vi "DBL-to-IEEE754.vi"(11 "Input_DBL":dbl(slide) scale=-20.0..20.0) -> (3 "Output_U8":u8[](array[numeric]))   [LabVIEW 2017]
panel:
  out "Array":bool[][](array[boolean])
  out "appended array":bool[](array[boolean])
  out "Sign":bool=TRUE
  out "Mantissa":bool[](array[boolean])=[TRUE, FALSE, FALSE, TRUE, FALSE, TRUE, FALSE, FALSE, FALSE, TRUE, TRUE, FALSE, FALSE, TRUE, TRUE, TRUE, FALSE, TRUE, TRUE, FALSE, TRUE, TRUE, FALSE]
  out "Exponent":bool[](array[boolean])=[TRUE, FALSE, FALSE, FALSE, FALSE, TRUE, FALSE, TRUE]
  out "Number":dbl=-101.10099792480469 format="%.12f"
  out "Exponent 2":dbl=6.0 format="%.2f"
  out "Mantissa 2":dbl=1.5797030925750732 format="%.8f"
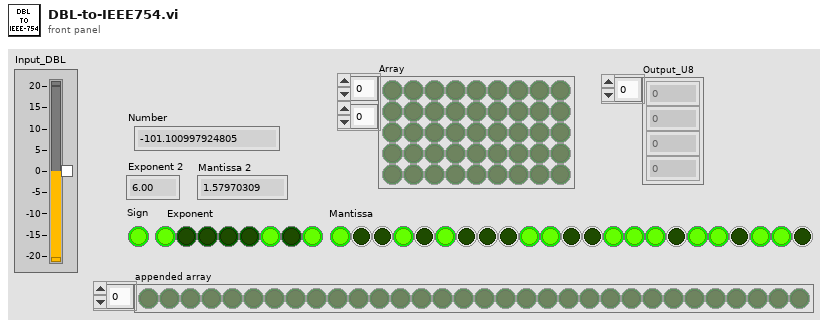
[diagram p1: front panel]
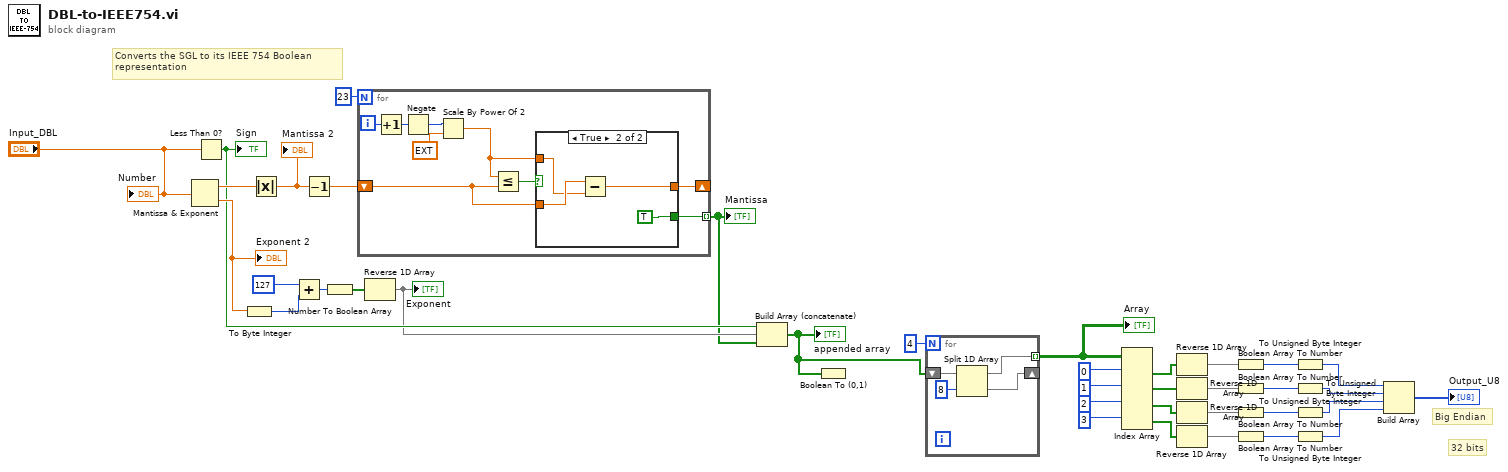
[diagram p0: block diagram]
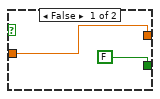
[diagram p2: hidden frame]
diagram:
  # "32 bits"
  # "Big Endian"
  # "Converts the SGL to its IEEE 754 Boolean \nrepresentation"
  n1 = Mantissa & Exponent(0:"Input_DBL") -> (1:w29:dbl, 2:w31:dbl)
  "Exponent 2" <- w31
  n2 = Less Than 0?(x="Input_DBL") -> (x < 0?=w28:bool)
  "Sign" <- w28
  n3 = To Byte Integer(number=w31) -> (8bit integer=w37:i8)
  n4 = Absolute Value(x=w29) -> (abs(x)=w30:dbl)
  "Mantissa 2" <- w30
  n5 = Add(x=i8 127, y=w37) -> (x+y=w36:i8)
  n6 = Decrement(x=w30) -> (x-1=w33:dbl)
  n7 = Number To Boolean Array(number=w36) -> (Boolean array=w35:bool[])
  n8 = for {
    N: 23 -> [_]
    shift-right: [w39] -> _
    shift-left: w33 -> [w41]
    tunnel: [w38] -> w26 mode=indexing
    i -> [w46]
    n9 = Increment(x=w46) -> (x+1=w45:i32)
    n10 = Negate(x=w45) -> (-x=w44:i32)
    n11 = Scale By Power Of 2(n=w44, x=ext 1.0) -> (x*2^n=w40:ext)
    n12 = Less Or Equal?(x=w40, y=w41) -> (x <= y?=w42:bool)
    n13 = case shown="True" w42 {
      tunnel: w41 -> [w47 w52]
      tunnel: w40 -> [_ w49]
      tunnel: [w47 w51] -> w39
      tunnel: [FALSE TRUE] -> w38
      frame False {
      }
      frame True {
        n14 = Subtract(x=w52, y=w49) -> (x-y=w51:ext)
      }
    }
  }
  "Mantissa" <- w26
  n15 = Reverse 1D Array(array=w35) -> (reversed array=w27:bool[])
  "Exponent" <- w27
  n16 = Build Array (concatenate)(w28, w27, w26) -> (w24:bool[])
  "appended array" <- w24
  n17 = Boolean To (0,1)(Boolean=w24) -> ()  [unwired: 1 out]
  n18 = for {
    N: 4 -> [_]
    shift-right: [w55] -> _
    shift-left: w24 -> [w56]
    tunnel: [w54] -> w23 mode=indexing
    n19 = Split 1D Array(array=w56, index=8) -> (first subarray=w54:bool[], second subarray=w55:bool[])
  }
  "Array" <- w23
  n20 = Index Array(array=w23, index (row) #1=0 ("disabled index (col)"), index (row) #2=1 ("index (col)"), index (row) #3=2 ("index (col)"), index (row) #4=3 ("index (col)")) -> (element #1=w4:bool[], element #2=w3:bool[], element #3=w2:bool[], element #4=w1:bool[])  [unwired: 4 in]
  n21 = Reverse 1D Array(array=w4) -> (reversed array=w8:bool[])
  n22 = Reverse 1D Array(array=w3) -> (reversed array=w7:bool[])
  n23 = Reverse 1D Array(array=w2) -> (reversed array=w6:bool[])
  n24 = Reverse 1D Array(array=w1) -> (reversed array=w5:bool[])
  n25 = Boolean Array To Number(Boolean array=w8) -> (number=w18:u32)
  n26 = Boolean Array To Number(Boolean array=w7) -> (number=w17:u32)
  n27 = Boolean Array To Number(Boolean array=w6) -> (number=w16:u32)
  n28 = Boolean Array To Number(Boolean array=w5) -> (number=w15:u32)
  n29 = To Unsigned Byte Integer(number=w18) -> (unsigned 8bit integer=w12:u8)
  n30 = To Unsigned Byte Integer(number=w17) -> (unsigned 8bit integer=w11:u8)
  n31 = To Unsigned Byte Integer(number=w16) -> (unsigned 8bit integer=w10:u8)
  n32 = To Unsigned Byte Integer(number=w15) -> (unsigned 8bit integer=w9:u8)
  n33 = Build Array(w12, w11, w10, w9) -> (→"Output_U8":u8[])
  "Number" <- "Input_DBL"
